vi "Find and Rejoin Devices.vi"(8 "error in":errorcluster, 11 "Generic Optimization in":refnum<class "Generic Optimization.lvclass">) -> (0 "error out":errorcluster, 3 "Generic Optimization out":refnum<class "Generic Optimization.lvclass">)   [LabVIEW 2018, in "Generic Optimization Actor.lvlib" / "Generic Optimization.lvclass"]
uses:
  Generic Optimization.lvclass
  C:/Users/Administrator/Desktop/2018LabVIEW EMS/EMS Generic Actor/EMS Generic/EMS Generic.lvclass
  C:/Users/Administrator/Desktop/2018LabVIEW EMS/Device Communication and Control Abstract Actor/Device Communication and Control Abstract/Device Communication and Control Abstract.lvclass
  EMS Generic Actor/EMS Generic/EMS Generic.lvclass/EMS Generic.ctl
  <vilib>/ORNL/CSEISMIC DDS/CSEISMIC DDS Base/Data Types/IED_Status.ctl
  <vilib>/ORNL/CSEISMIC DDS/CSEISMIC DDS Base/Data Types/Controls/DeviceID.ctl
  <vilib>/ORNL/CSEISMIC DDS/CSEISMIC DDS Base/Data Types/Controls/Timestamp.ctl
  <vilib>/ORNL/CSEISMIC DDS/CSEISMIC DDS Base/Data Types/Controls/Generation Mode.ctl
  <vilib>/ORNL/CSEISMIC DDS/CSEISMIC DDS Base/Data Types/DER_VF.ctl
  <vilib>/ActorFramework/Actor/Actor.lvclass/Actor.ctl
  Device Communication and Control Abstract Actor/Device Communication and Control Abstract/Device Communication and Control Abstract.lvclass/Device Communication and Control Abstract.ctl
  Device Communication and Control Abstract Actor/Device Communication and Control Abstract Messages/Set DER VF Msg/Set DER VF Msg.lvclass/Set DER VF Msg.ctl
  <vilib>/ActorFramework/Message Enqueuer/Message Enqueuer.lvclass/Message Enqueuer.ctl
  Device Communication and Control Abstract Actor/Device Communication and Control Abstract Messages/Set DER VF Msg/Send Set DER VF.vi
  <vilib>/ActorFramework/Actor/Read Caller Enqueuer.vi
  <vilib>/ActorFramework/Message Enqueuer/Enqueue.vi
  Device Communication and Control Abstract Actor/Device Communication and Control Abstract/Device Communication and Control Abstract.lvclass
  C:/Program Files (x86)/National Instruments/LabVIEW 2018/vi.lib/ActorFramework/Actor/Actor.lvclass
  Device Communication and Control Abstract Actor/Device Communication and Control Abstract Messages/Set DER VF Msg/Set DER VF Msg.lvclass
  C:/Program Files (x86)/National Instruments/LabVIEW 2018/vi.lib/ActorFramework/Message/Message.lvclass
  <vilib>/ActorFramework/Message Priority Queue/Priority Enqueue.vi
  <vilib>/ORNL/CSEISMIC DDS/CSEISMIC DDS Base/CSEISMIC DDS.lvclass
  Utilities/Status Messaging.llb/Status Messaging.lvlib
  EMS Generic Actor/EMS Generic/EMS Generic.lvclass
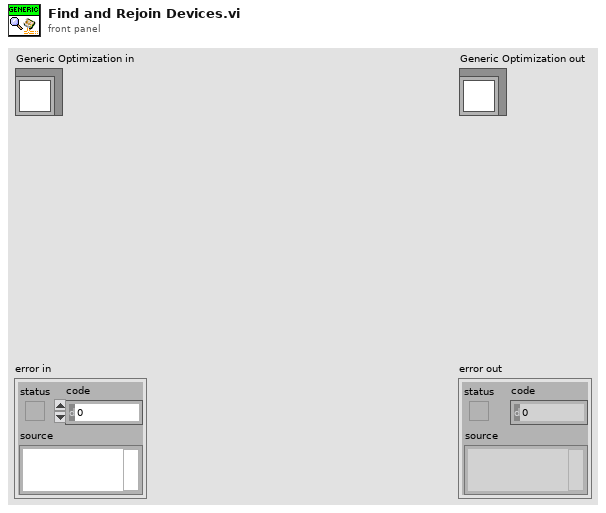
[diagram p1: front panel]
types:
  T1 = typedef "CSEISMIC DDS.lvlib/CSEISMIC DDS.lvclass/DER_VF.ctl" = cluster{"DeviceID":T2}
  T2 = typedef "CSEISMIC DDS.lvlib/CSEISMIC DDS.lvclass/DeviceID.ctl" = string
  T3 = typedef "CSEISMIC DDS.lvlib/CSEISMIC DDS.lvclass/IED_Status.ctl" = cluster{"DeviceID":T2, "Timestamp":T4, "MicrogridID":u8, "Active":bool, "Inactive":bool, "Error":i32, "Fault":bool, "ErrorString":string}
  T4 = typedef "CSEISMIC DDS.lvlib/CSEISMIC DDS.lvclass/Timestamp.ctl" = cluster{"Seconds":u64, "Remainder":u64}
  T5 = typedef "CSEISMIC DDS.lvlib/CSEISMIC DDS.lvclass/Generation Mode.ctl" = enum32{"Invalid", "PQ", "Droop", "PV", "PF", "VF"}
  T6 = typedef "EMS Generic Actor.lvlib/EMS Generic.lvclass/Data Type DVRs.ctl" = cluster{"IED_Status":refnum<data-value>, "IED_Status_0":refnum<data-value>, "DER_Measurement":refnum<data-value>, "DER_Info":refnum<data-value>, "DER_Status":refnum<data-value>, "ES_Measurement":refnum<data-value>, "ES_Info":refnum<data-value>, "PV_Info":refnum<data-value>, "SmartRelay_Info":refnum<data-value>, "SmartRelay_Measurement":refnum<data-value>, "Meter_Info":refnum<data-value>, "Meter_Measurement":refnum<data-value>, "HVAC_Status":refnum<data-value>, "HVAC_Measurement":refnum<data-value>, "PriceData_RealTime":refnum<data-value>, "PriceData_Demand":refnum<data-value>, "PriceData_Energy":refnum<data-value>, "ForecastData_Long":refnum<data-value>, "ForecastData_Short":refnum<data-value>, "DER_Control":refnum<data-value>, "DER_SetPointF":refnum<data-value>, "DER_SetPointP":refnum<data-value>, "DER_SetPointQ":refnum<data-value>, "DER_SetPointPF":refnum<data-value>, "DER_SetPointV":refnum<data-value>, "PV_setCurtailment":refnum<data-value>, "PV_setRampRate":refnum<data-value>, "Relay_Control":refnum<data-value>, "Load_Control":refnum<data-value>, "HVAC_Control":refnum<data-value>, "Generator_Info":refnum<data-value>, "ForecastData_Long_Backup":refnum<data-value>, "PriceData_RealTime_Backup":refnum<data-value>}
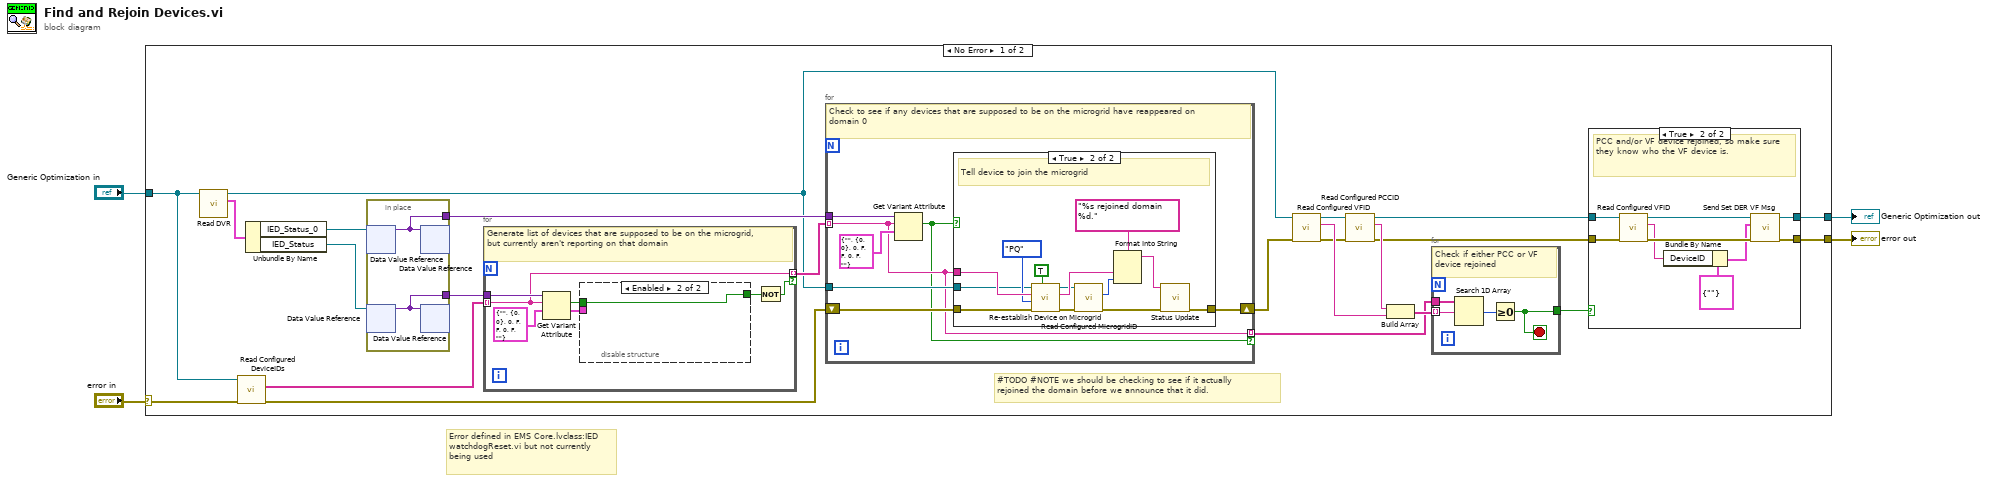
[diagram p0: block diagram]
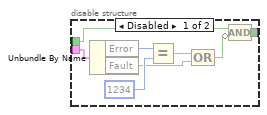
[diagram p3: hidden frame]
diagram:
  # "Error defined in EMS Core.lvclass:IED watchdogReset.vi but not currently being used"
  n1 = case shown="No Error" "error in" {
    selector: "error in" -> [w22 w82]
    tunnel: [w7 w82] -> w3
    tunnel: [w5 w81] -> w1
    tunnel: "Generic Optimization in" -> [w19 w81]
    frame No Error {
      # "#TODO #NOTE we should be checking to see if it actually rejoined the domain before we announce that it did."
      n2 = call "Read DVR.vi"("EMS Generic in"=w19) -> ("DVR"=w18:T6, "EMS Generic out"=w6:refnum<class "Generic Optimization.lvclass">)  [unwired: 9 in]
      n3 = call "Read Configured DeviceIDs.vi"("error in"=w22, "EMS Generic in"=w19) -> ("error out"=w21:errorcluster, "DeviceIDs"=w20:T2[])  [unwired: 7 in, 1 out]
      n4 = Unbundle By Name(w18) -> ("IED_Status_0"=w23:refnum<data-value>, "IED_Status"=w24:refnum<data-value>)
      n5 = in-place {
        in-place-border: [w44] -> w25
        in-place-border: [w43] -> w26
        n6 = in-place-dvr #1(w23) -> (w43:variant)  [unwired: 1 out]
        n7 = in-place-dvr #2(w24) -> (w44:variant)  [unwired: 1 out]
        n8 = in-place-dvr #1(w43) -> ()  [unwired: 2 out]
        n9 = in-place-dvr #2(w44) -> ()  [unwired: 2 out]
      }
      n10 = for {
        tunnel: w20 -> [w47] mode=indexing
        tunnel: w25 -> [w51]
        tunnel: [w47] -> w27 mode=indexing if=w46
        # "Generate list of devices that are supposed to be on the microgrid, but currently aren't reporting on that domain"
        n11 = Get Variant Attribute(Variant=w51, name=w47, default value (empty Variant)=T3 {"DeviceID"="", "Timestamp"={"Seconds"=0, "Remainder"=0}, "MicrogridID"=0, "Active"=FALSE, "Inactive"=FALSE, "Error"=0, "Fault"=FALSE, "ErrorString"=""} ("IED_Status")) -> (found=w48:bool, value=w49:T3)  [unwired: 1 in, 2 out]
        n12 = disable-structure shown="Enabled" {
          disable-tunnel: w49 -> [w59 _]
          disable-tunnel: w48 -> [w57 w60]
          disable-tunnel: [w56 w60] -> w45
          frame Disabled {
            n13 = Unbundle By Name(w59) -> ("Error"=w54:i32, "Fault"=w52:bool)
            n14 = Equal?(x=w54, y=1234) -> (x = y?=w55:bool)
            n15 = Compound Arithmetic op=OR(w55, w52) -> (w53:bool)
            n16 = Compound Arithmetic op=AND(w57, invert w53) -> (w56:bool)
          }
          frame Enabled {
          }
        }
        n17 = Not(x=w45) -> (.not. x?=w46:bool)
      }
      n18 = for {
        tunnel: w26 -> [w67]
        tunnel: w27 -> [w62] mode=indexing
        tunnel: w6 -> [w65]
        shift-right: [w63] -> w17
        shift-left: w21 -> [w64]
        tunnel: [w62] -> w11 mode=indexing if=w61
        # "Check to see if any devices that are supposed to be on the microgrid have reappeared on domain 0"
        n19 = Get Variant Attribute(Variant=w67, name=w62, default value (empty Variant)=T3 {"DeviceID"="", "Timestamp"={"Seconds"=0, "Remainder"=0}, "MicrogridID"=0, "Active"=FALSE, "Inactive"=FALSE, "Error"=0, "Fault"=FALSE, "ErrorString"=""} ("IED_Status")) -> (found=w61:bool)  [unwired: 1 in, 3 out]
        n20 = case shown="True" w61 {
          tunnel: w62 -> [_ w75]
          tunnel: w65 -> [_ w69]
          tunnel: w64 -> [w68 w72]
          tunnel: [w68 w76] -> w63
          frame False {
          }
          frame True {
            # "Tell device to join the microgrid"
            n21 = call "Re-establish Device on Microgrid.vi"("Activate"=TRUE, "error in"=w72, "Mode"=Generation_Mode."PQ", "DeviceID"=w75, "Generic Optimization in"=w69) -> ("error out"=w71:errorcluster, "Generic Optimization out"=w70:refnum<class "Generic Optimization.lvclass">)  [unwired: 5 in]
            n22 = call "Read Configured MicrogridID.vi"("error in"=w71, "EMS Generic in"=w70) -> ("error out"=w77:errorcluster, "Microgrid ID"=w80:u8)  [unwired: 7 in, 1 out]
            n23 = Format Into String(format string="%s rejoined domain %d.", w75, w80) -> (resulting string=w78:string)  [unwired: 2 in, 1 out]
            n24 = call "Status Update.vi"("error in"=w77, "Status Update"=w78) -> ("error out"=w76:errorcluster)  [unwired: 8 in, 1 out]
          }
        }
      }
      n25 = call "Read Configured VFID.vi"("error in"=w17, "EMS Generic in"=w6) -> ("error out"=w13:errorcluster, "VFID"=w14:T2, "EMS Generic out"=w16:refnum<class "Generic Optimization.lvclass">)  [unwired: 7 in]
      n26 = call "Read Configured PCCID.vi"("error in"=w13, "EMS Generic in"=w16) -> ("error out"=w9:errorcluster, "PCCID"=w15:T2, "EMS Generic out"=w8:refnum<class "Generic Optimization.lvclass">)  [unwired: 7 in]
      n27 = Build Array(w15, w14) -> (w12:T2[])
      n28 = for {
        tunnel: w12 -> [w41] mode=indexing
        tunnel: w11 -> [w42]
        tunnel: [w39] -> w10
        stop <- w39 stop-if-true
        # "Check if either PCC or VF device rejoined"
        n29 = Search 1D Array(1D array=w42, element=w41) -> (index of element=w40:i32)  [unwired: 1 in]
        n30 = Greater Or Equal To 0?(x=w40) -> (x >= 0?=w39:bool)
      }
      n31 = case shown="True" w10 {
        tunnel: w9 -> [w29 w37]
        tunnel: w8 -> [w28 w38]
        tunnel: [w29 w30] -> w7
        tunnel: [w28 w31] -> w5
        frame False {
          # "The device that rejoined is not the VF device or the PCC, so it doesn't matter if they know who the VF device is.  Do nothing."
        }
        frame True {
          # "PCC and/or VF device rejoined, so make sure they know who the VF device is."
          n32 = call "Read Configured VFID.vi"("error in"=w37, "EMS Generic in"=w38) -> ("error out"=w35:errorcluster, "VFID"=w33:T2, "EMS Generic out"=w34:refnum<class "Generic Optimization.lvclass">)  [unwired: 7 in]
          n33 = Bundle By Name(cluster=T1 {"DeviceID"=""} ("DER_VF"), "DeviceID"=w33) -> (w32:T1)
          n34 = call "Send Set DER VF Msg.vi"("error in"=w35, "DER_VF"=w32, "SCADA Sub Abstract in"=w34) -> ("error out"=w30:errorcluster, "dup SCADA Sub Abstract"=w31:refnum<class "Generic Optimization.lvclass">)  [unwired: 7 in]
        }
      }
    }
    frame Error {
    }
  }
  "error out" <- w3
  "Generic Optimization out" <- w1
